vi "UserDefined Smybol AE.vi"(7 "Mode":enum16{"Set", "Get", "Restore"}(ring), 8 "错误输入":errorcluster, 9 "Index":i32, 10 "图像":T1, 11 "Mlistbox Ref":refnum<vi>) -> (0 "错误输出":errorcluster, 2 "Image":T1 caption="图像", 3 "Mlistbox Ref Dup":refnum<vi>)   [LabVIEW 2012, in "Mlistbox Tools.lvlib"]
uses:
  Mlistbox Tools.lvlib
  <vilib>/picture/picture.llb/imagedata.ctl
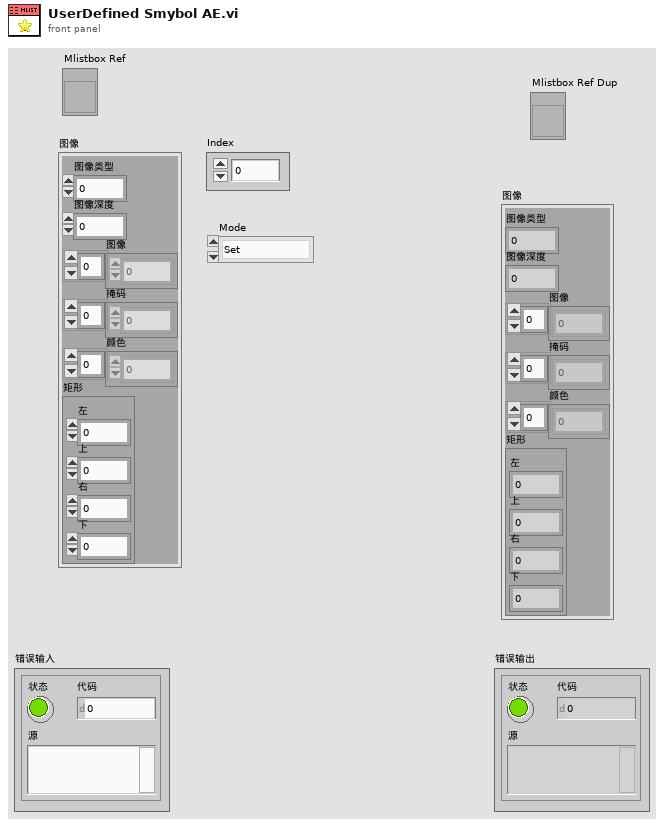
[diagram p1: front panel]
types:
  T1 = typedef "imagedata.ctl" = cluster{"image type":i32, "image depth":i32, "image":u8[], "mask":u8[], "colors":u32[], "Rectangle":cluster{"left":i16, "top":i16, "right":i16, "bottom":i16}}
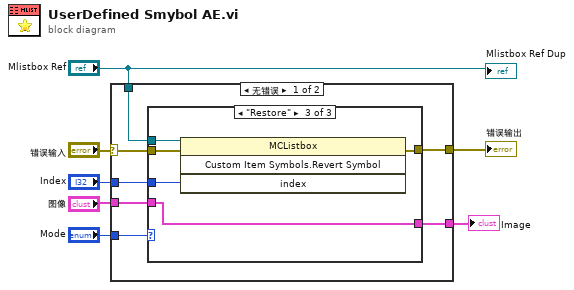
[diagram p0: block diagram]
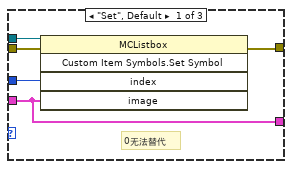
[diagram p2: hidden frame]
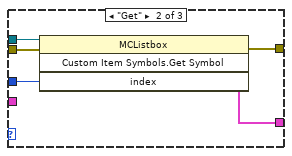
[diagram p3: hidden frame]
diagram:
  n1 = case shown="无错误" "错误输入" {
    selector: "错误输入" -> [w13 w30]
    tunnel: [w12 w30] -> w1
    tunnel: "Mlistbox Ref" -> [w14 _]
    tunnel: "Index" -> [w11 _]
    tunnel: [w10 _] -> w5
    tunnel: "Mode" -> [w9 _]
    tunnel: "图像" -> [w8 _]
    frame No Error {
      n2 = case shown="\"Restore\"" w9 {
        tunnel: w14 -> [w18 w24 w28]
        tunnel: w13 -> [w19 w23 w29]
        tunnel: [w17 w22 w27] -> w12
        tunnel: w11 -> [w16 w21 w25]
        tunnel: [w15 w20 w26] -> w10
        tunnel: w8 -> [w15 _ w26]
        frame "Set", Default {
          # "0无法替代"
          n3 = invoke class="MCListbox" method="Custom Item Symbols.Set Symbol"(reference=w18, error in=w19, "index"=w16, "image"=w15) -> (error out=w17:errorcluster)  [unwired: 1 in, 4 out]
        }
        frame "Get" {
          n4 = invoke class="MCListbox" method="Custom Item Symbols.Get Symbol"(reference=w24, error in=w23, "index"=w21) -> (error out=w22:errorcluster, "Custom Item Symbols:Get Symbol"=w20:T1)  [unwired: 1 in, 2 out]
        }
        frame "Restore" {
          n5 = invoke class="MCListbox" method="Custom Item Symbols.Revert Symbol"(reference=w28, error in=w29, "index"=w25) -> (error out=w27:errorcluster)  [unwired: 1 in, 3 out]
        }
      }
    }
    frame Error {
    }
  }
  "错误输出" <- w1
  "Image" <- w5
  "Mlistbox Ref Dup" <- "Mlistbox Ref"
